vi "SetParam.vi"(8 "error in (no error)":errorcluster caption="entrée d'erreur (pas d'erreur)", 10 "make_gaussian_quantiles":T1={"mean"=[-1.0], "cov "=1.0, "n_samples"=100, "n_features"=2, "n_classes"=3, "shuffle"=TRUE, "random_state"=-1, "Returns"="X"} {"random_state" min=-1; "n_classes" min=1; "n_features" min=1; "n_samples" min=1}, 11 "Gaussian_Quantiles.lvclass":refnum<class "Gaussian_Quantiles.lvclass">) -> (0 "error out":errorcluster caption="sortie d'erreur", 3 "Gaussian_Quantiles.lvclass":refnum<class "Gaussian_Quantiles.lvclass">)   [LabVIEW 2020, in "Gaussian_Quantiles.lvclass"]
doc: "Set Parameters"
uses:
  Gaussian_Quantiles.lvclass
  Gaussian_Quantiles.lvclass/Gaussian_Quantiles.ctl
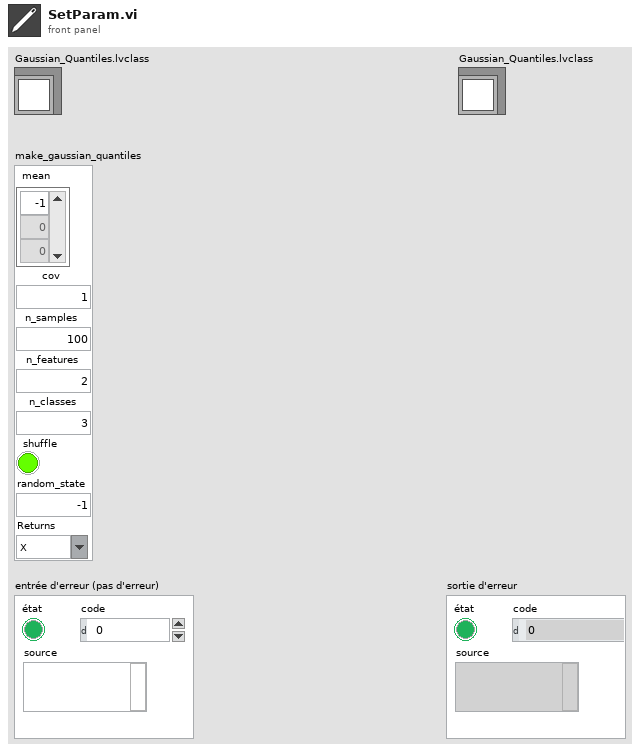
[diagram p1: front panel]
types:
  T1 = cluster{"mean":dbl[], "cov ":dbl, "n_samples":u32, "n_features":u32, "n_classes":u32, "shuffle":bool, "random_state":i32, "Returns":string}
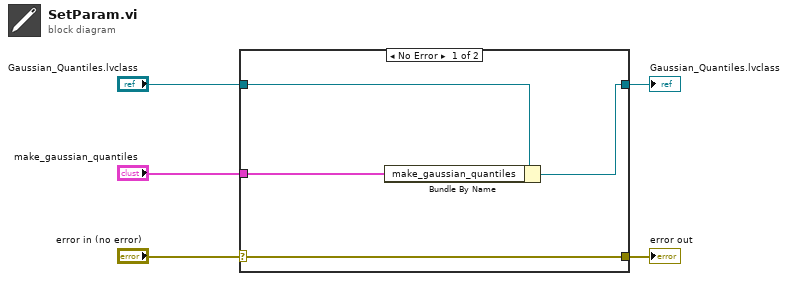
[diagram p0: block diagram]
diagram:
  n1 = case shown="No Error" "error in (no error)" {
    selector: "error in (no error)" -> [w9 w10]
    tunnel: [w9 w10] -> w4
    tunnel: [w7 w11] -> w2
    tunnel: "Gaussian_Quantiles.lvclass" -> [w8 w11]
    tunnel: "make_gaussian_quantiles" -> [w6 _]
    frame No Error {
      n2 = Bundle By Name(cluster=w8, "make_gaussian_quantiles"=w6) -> (w7:refnum<class "Gaussian_Quantiles.lvclass">)
    }
    frame Error {
    }
  }
  "error out" <- w4
  "Gaussian_Quantiles.lvclass" <- w2
